vi "Generate Async Msg Event.vi"(6 "bypass (F)":bool, 7 "AdHoc Msg (\"\")":string, 8 "error in (no error)":errorcluster, 9 "vData":variant, 10 "AsyncMsg":T1, 11 "Log_Engine in":refnum<class "Log_Engine.lvclass">) -> (0 "error out":errorcluster, 3 "Log_Engine out":refnum<class "Log_Engine.lvclass">)   [LabVIEW 2019, in "Log_Engine.lvclass"]
doc: "Developed by Kevin Thompson\nkevin@thompsonengineering.net\n\nCopyright 2018\nThompson Engineering, LLC"
uses:
  Log_Engine.lvclass
  Common/DataTypes/TD Async CmdMsg EventData--cluster.ctl
  DataTypes/AsynMsg_Log_Engine--enum.ctl
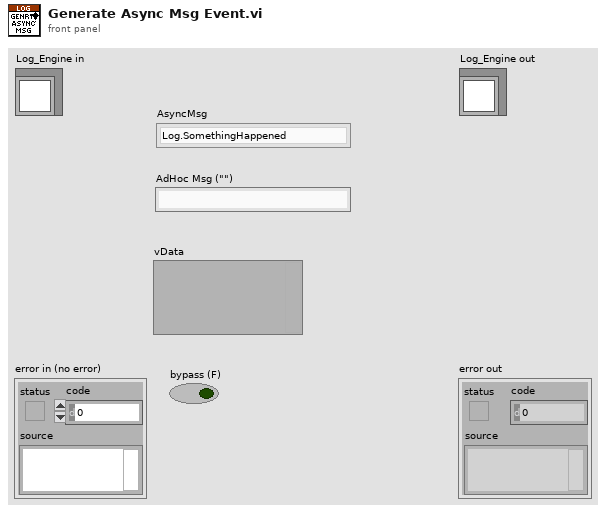
[diagram p1: front panel]
types:
  T1 = typedef "Log_Engine.lvclass/AsynMsg_Log_Engine--enum.ctl" = enum16{"Log.SomethingHappened"}
  T2 = typedef "TD Async CmdMsg EventData--cluster.ctl" = cluster{"Time Stamp":timestamp, "CmdMsg":string, "vData":variant}
  T3 = typedef "Log_Engine.lvclass/Public Events--cluster.ctl" = cluster{"Log_Engine.AsyncCmd Event":refnum<user-event>, "Log_Engine.AsyncMsg Event":refnum<user-event>, "stop process":refnum<user-event>, "Log_Engine.LogStateChg Ev":refnum<user-event>, "Log_Engine.TDMSStateChg Ev":refnum<user-event>}
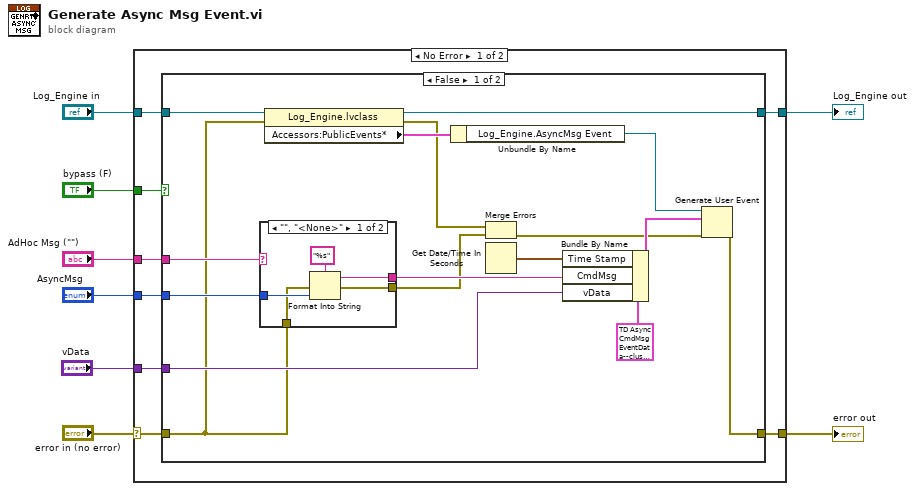
[diagram p0: block diagram]
diagram:
  n1 = case shown="No Error" "error in (no error)" {
    selector: "error in (no error)" -> [w10 w43]
    tunnel: [w16 w43] -> w3
    tunnel: [w11 w42] -> w7
    tunnel: "Log_Engine in" -> [w12 w42]
    tunnel: "AsyncMsg" -> [w14 _]
    tunnel: "vData" -> [w15 _]
    tunnel: "AdHoc Msg (\"\")" -> [w13 _]
    tunnel: "bypass (F)" -> [w9 _]
    frame No Error {
      n2 = case shown="False" w9 {
        tunnel: [w32 w40] -> w16
        tunnel: w15 -> [w27 _]
        tunnel: w14 -> [w25 _]
        tunnel: w13 -> [w24 _]
        tunnel: w12 -> [w22 w41]
        tunnel: [w21 w41] -> w11
        tunnel: w10 -> [w17 w40]
        frame False {
          n3 = case shown="\"\", \"<None>\"" w24 {
            selector: w24 -> [_ w38]
            tunnel: w25 -> [w36 _]
            tunnel: [w35 w38] -> w28
            tunnel: w17 -> [w34 w39]
            tunnel: [w33 w39] -> w26
            frame "", "<None>" {
              n4 = Format Into String(format string="%s", error in=w34, w36) -> (resulting string=w35:string, error out=w33:errorcluster)  [unwired: 1 in]
            }
            frame Default {
            }
          }
          n5 = property class="Log_Engine.lvclass"(reference=w22, error in=w17) -> (reference out=w21:refnum<class "Log_Engine.lvclass">, error out=w18:errorcluster, "Accessors:PublicEvents*"=w23:T3)
          n6 = Unbundle By Name(w23) -> ("Log_Engine.AsyncMsg Event"=w20:refnum<user-event>)
          n7 = Merge Errors(w18, w26) -> (w19:errorcluster)
          n8 = Get Date/Time In Seconds() -> (seconds since 1Jan1904=w29:timestamp)
          n9 = Bundle By Name(cluster=T2 {"Time Stamp"=timestamp(0 s since 1904-01-01), "CmdMsg"="", "vData"=variant} ("Async EvData"), "Time Stamp"=w29, "CmdMsg"=w28, "vData"=w27) -> (w31:T2)
          n10 = Generate User Event(user event=w20, event data cluster=w31, error in=w19) -> (error out=w32:errorcluster)  [unwired: 1 in, 1 out]
        }
        frame True {
        }
      }
    }
    frame Error {
    }
  }
  "error out" <- w3
  "Log_Engine out" <- w7
